vi "Save Test Result.vi"(8 "error in (no error)":errorcluster, 10 "Report.lvclass":refnum<class "Report.lvclass">, 11 "Test Step in":refnum<class "Test Step.lvclass">) -> (0 "error out":errorcluster, 3 "Test Step out":refnum<class "Test Step.lvclass">)   [LabVIEW 2021, in "Sequence Engine.lvlib" / "Test Step.lvclass"]
uses:
  Test Step.lvclass
  Test Step.lvclass/Test Step.ctl
  PPLs/Report.lvlibp/Classes/Report/Report.lvclass
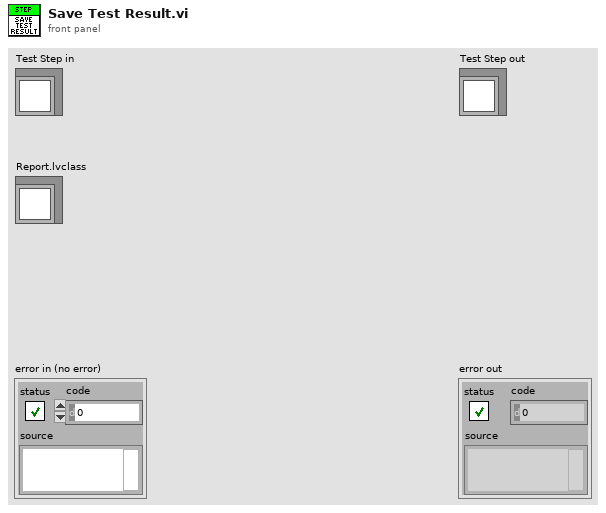
[diagram p1: front panel]
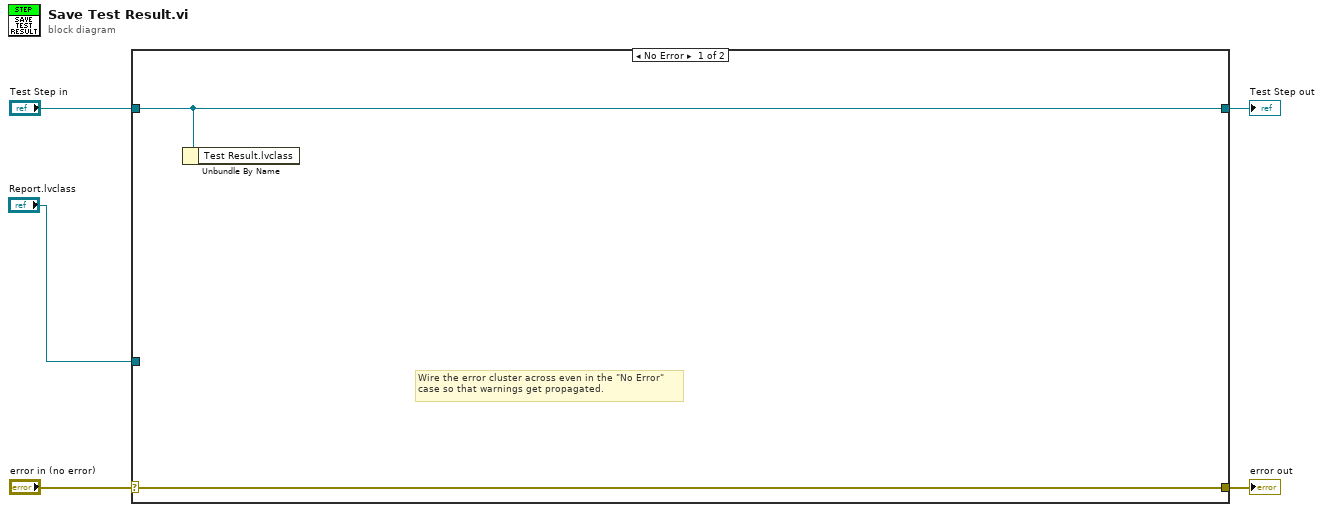
[diagram p0: block diagram]
diagram:
  n1 = case shown="No Error" "error in (no error)" {
    selector: "error in (no error)" -> [w6 w9]
    tunnel: [w6 w9] -> w4
    tunnel: [w7 w8] -> w2
    tunnel: "Test Step in" -> [w7 w8]
    tunnel: "Report.lvclass" -> [_ _]
    frame No Error {
      # "Wire the error cluster across even in the \"No Error\"\ncase so that warnings get propagated."
      n2 = Unbundle By Name(w7) -> ()  [unwired: 1 out]
    }
    frame Error {
    }
  }
  "error out" <- w4
  "Test Step out" <- w2
